vi "subSave_Img2Tiff.vi"(5 "Open file dialog? (F)":bool, 7 "Save Text file? (F)":bool, 8 "Error in (no error)":errorcluster, 9 "text":string, 10 "Image":u16[][](graph)=array512x512[262144 elements], 11 "File path/name":path=path "C:/Peng/Data") -> (0 "Error out":errorcluster, 3 "Cancel or not?":bool)   [LabVIEW 2015]
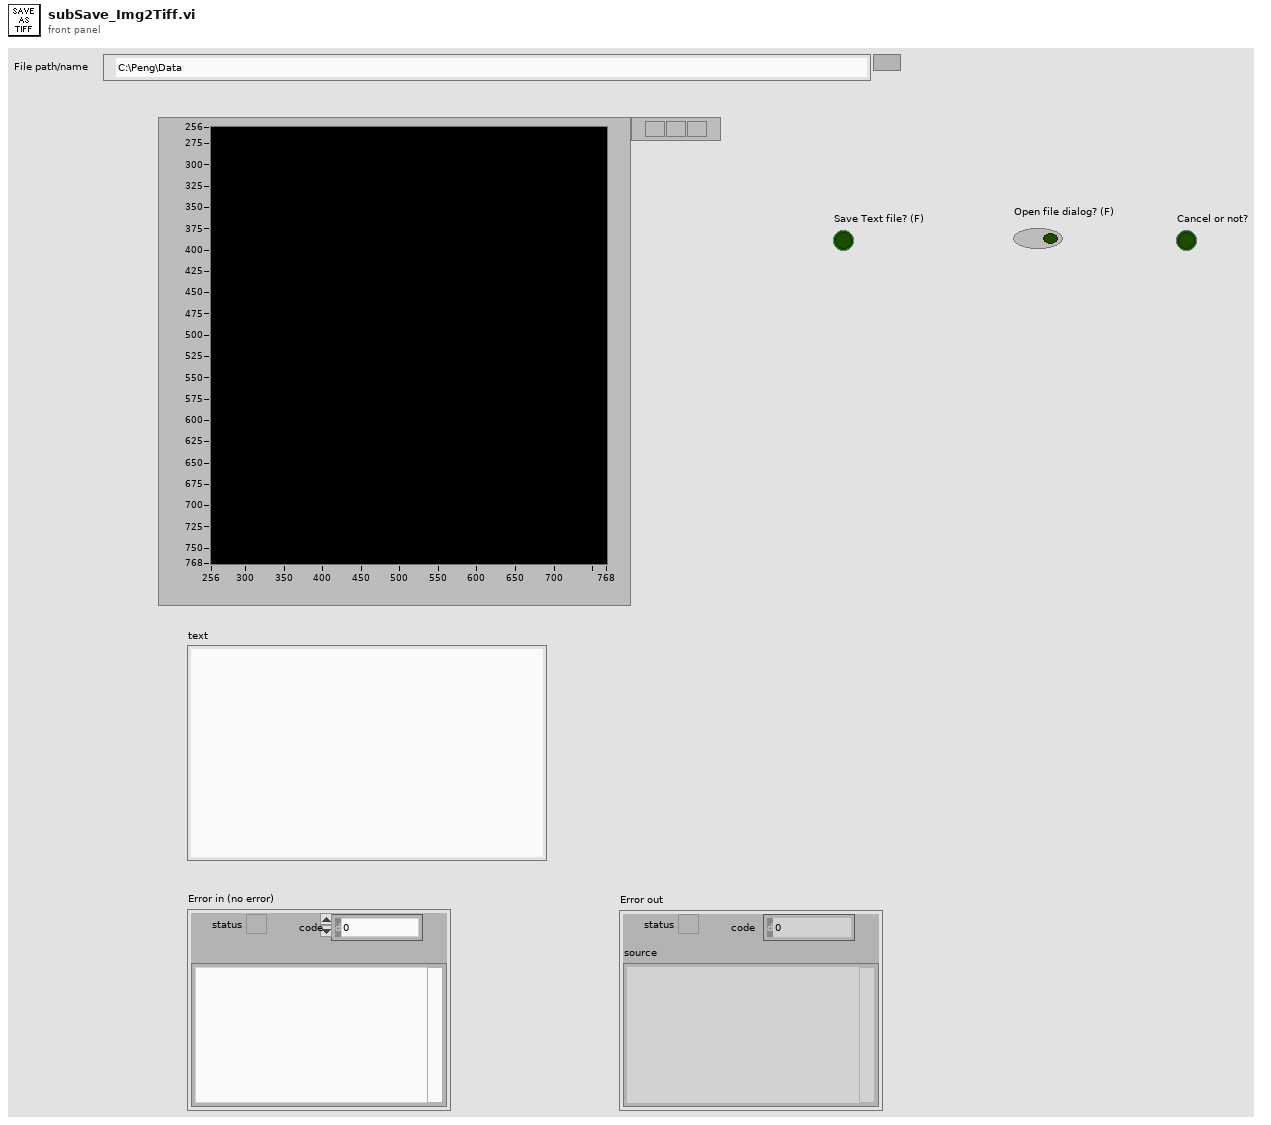
[diagram p1: front panel]
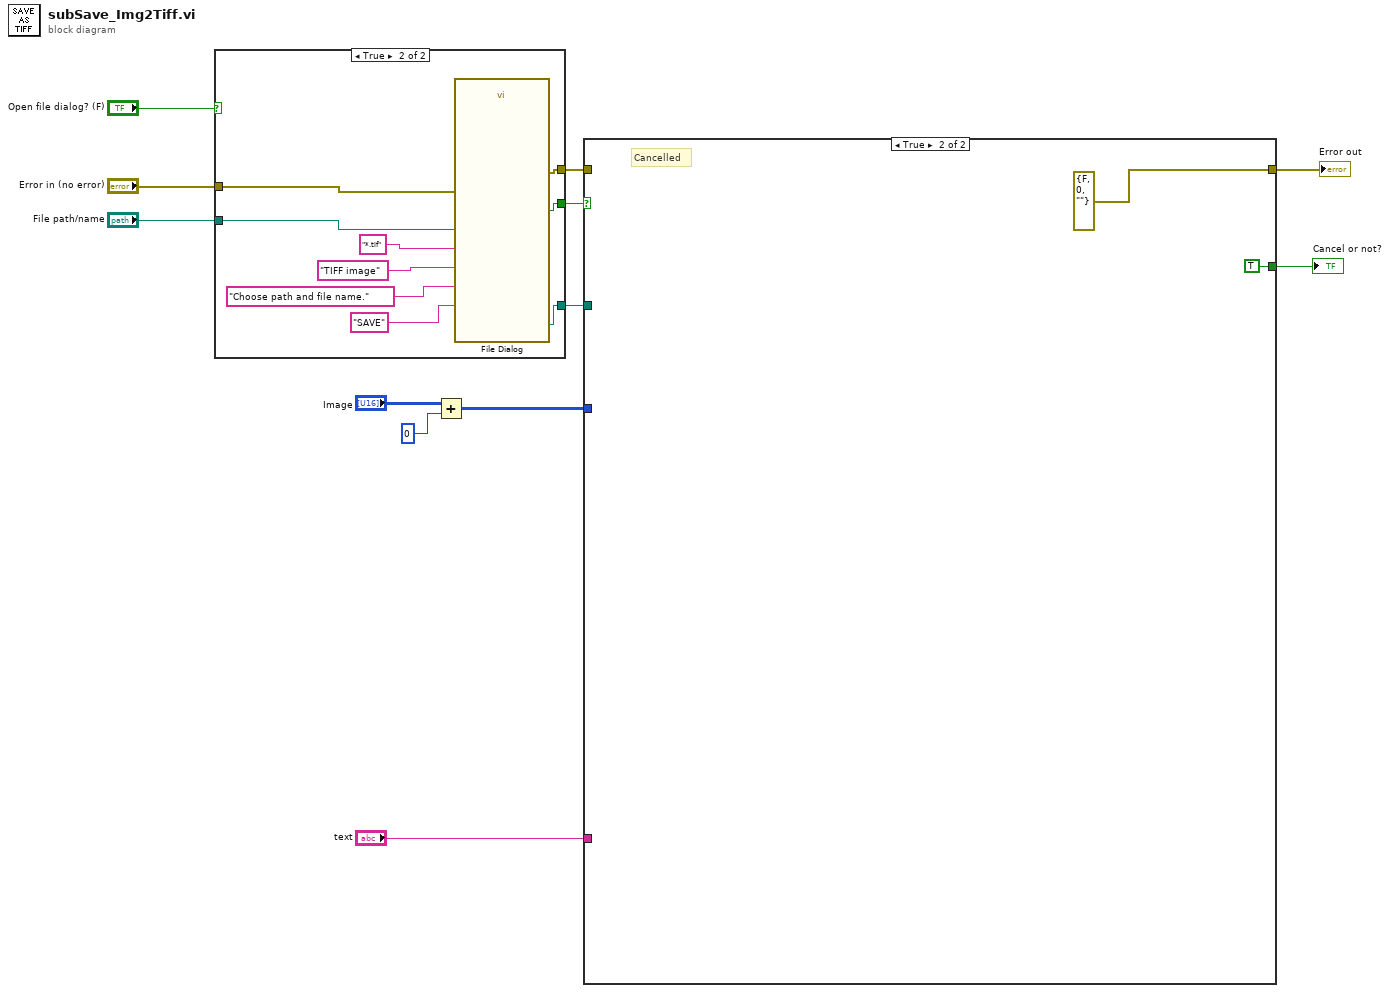
[diagram p0: block diagram]
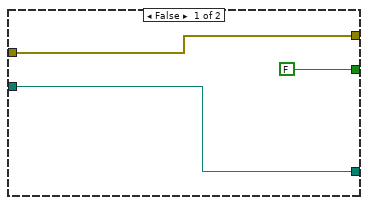
[diagram p2: hidden frame]
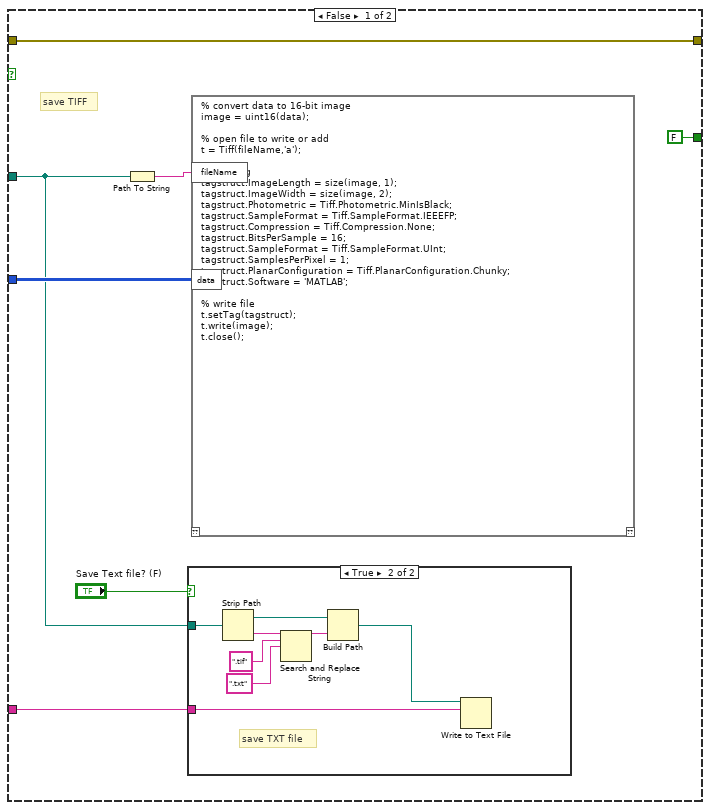
[diagram p3: hidden frame]
diagram:
  n1 = case shown="True" "Open file dialog? (F)" {
    tunnel: [FALSE ("cancelled") w20] -> w12
    tunnel: [w15 w19] -> w11
    tunnel: [w14 w18] -> w10
    tunnel: "File path/name" -> [w15 w17]
    tunnel: "Error in (no error)" -> [w14 w16]
    frame False {
    }
    frame True {
      n2 = call "File Dialog"("start path"=w17, "prompt"="Choose path and file name.", "button label"="SAVE", "error in"=w16, "pattern (all files)"="*.tif" ("default name"), "pattern label"="TIFF image" ("default name")) -> ("selected path"=w19:path, "cancelled"=w20:bool, "error out"=w18:errorcluster)  [unwired: 6 in, 1 out]
    }
  }
  n3 = Add(x="Image", y=0) -> (x+y=w5:i32[][])
  n4 = case shown="True" w12 {
    tunnel: w5 -> [w30 _]
    tunnel: w11 -> [w26 _]
    tunnel: "text" -> [w29 _]
    tunnel: w10 -> [w28 _]
    tunnel: [w28 errorcluster {"status"=FALSE, "code"=0, "source"=""} ("camera \ninitialization\nerror")] -> w8
    tunnel: [FALSE ("Cancel or not?") TRUE ("Cancel or not?")] -> w1
    frame False {
      # "save TIFF"
      n5 = Path To String(path=w26) -> (string=w31:string)
      n6 = case shown="True" "Save Text file? (F)" {
        tunnel: w26 -> [_ w34]
        tunnel: w29 -> [_ w33]
        frame False {
        }
        frame True {
          # "save TXT file"
          n7 = Strip Path(path=w34) -> (stripped path=w38:path, name=w35:string)
          n8 = Search and Replace String(input string=w35, search string=".tif", replace string=".txt" ("replace string (\"\")")) -> (result string=w39:string)  [unwired: 5 in, 3 out]
          n9 = Build Path(base path=w38, name or relative path=w39) -> (appended path=w32:path)
          n10 = Write to Text File(file (use dialog)=w32, text=w33) -> ()  [unwired: 2 in, 3 out]
        }
      }
      n11 = script code="% convert data to 16-bit image\nimage = uint16(data);\n\n% open file to write or add\nt = Tiff(fileName,'a');\n\n% edit tag\ntagstruct.ImageLength = size(image, 1);\ntagstruct.ImageWidth = size(image, 2);\ntagstruct.Photometric = Tiff.Photometric.MinIsBlack;\ntagstruct.SampleFormat = Tiff.SampleFormat.IEEEFP;\ntagstruct.Compression = Tiff.Compression.None;\ntagstruct.BitsPerSample = 16;\ntagstruct.SampleFormat = Tiff.SampleFormat.UInt;\ntagstruct.SamplesPerPixel = 1;\ntagstruct.PlanarConfiguration = Tiff.PlanarConfiguration.Chunky;\ntagstruct.Software = 'MATLAB';\n\n% write file\nt.setTag(tagstruct);\nt.write(image);\nt.close();"("fileName"=w31, "data"=w30) -> ()  [unwired: 1 in, 1 out]
    }
    frame True {
      # "Cancelled"
    }
  }
  "Error out" <- w8
  "Cancel or not?" <- w1
